vi "Result_Test.vi"(8 "error in (no error)":errorcluster caption="entrée d'erreur (pas d'erreur)", 11 "Delay en entrée":refnum<class "Enter_SN_PCRE.lvclass">) -> (0 "error out":errorcluster caption="sortie d'erreur", 3 "Delay en sortie":refnum<class "Enter_SN_PCRE.lvclass">)   [LabVIEW 2020, in "Library Test.lvlib" / "Enter_SN_PCRE.lvclass"]
uses:
  Enter_SN_PCRE.lvclass
  C:/Users/ngarcin/OneDrive - Altyor/Standard TB/Suite TB45/Class/Test/Test (Default)/Test (Default).lvclass
  Commun VI/TypeDef/Variable Printable.ctl
  Creation_SN/Creation_SN Database (Default)/Creation_SN Database (Default).lvclass
  Test_Without_Instr/Test_Without_Inst.lvclass
  Commun VI/Library Commun.lvlib
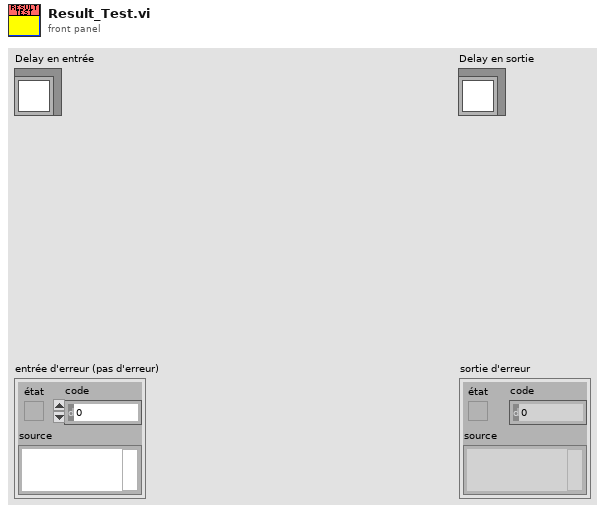
[diagram p1: front panel]
types:
  T1 = typedef "Variable Printable.ctl" = string
  T2 = enum16{"Get Variable", "Get All Variables", "Set Variable", "Delete Variable", "Delete All Variable"}
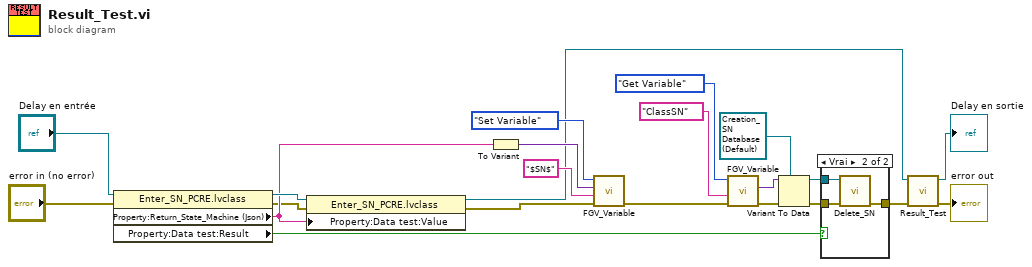
[diagram p0: block diagram]
diagram:
  n1 = property class="Enter_SN_PCRE.lvclass"(reference="Delay en entrée", error in="error in (no error)") -> (reference out=w15:refnum<class "Enter_SN_PCRE.lvclass">, error out=w12:errorcluster, "Property:Return_State_Machine (Json)"=w14:string, "Property:Data test:Result"=w1:bool)
  n2 = property class="Enter_SN_PCRE.lvclass"(reference=w15, error in=w12, "Property:Data test:Value"=w14) -> (reference out=w13:refnum<class "Enter_SN_PCRE.lvclass">, error out=w11:errorcluster)
  n3 = To Variant(anything=w14) -> (Variant=w17:variant)
  n4 = call "FGV_Variable.vi"("error in (no error)"=w11, "Variable"="$SN$" ("Name"), "Data In"=w17, "Function"=T2."Set Variable") -> ("error out"=w8:errorcluster)  [unwired: 5 in, 2 out]
  n5 = call "FGV_Variable.vi"("error in (no error)"=w8, "Variable"=T1 "ClassSN", "Function"=T2."Get Variable") -> ("error out"=w6:errorcluster, "Data Out"=w7:variant)  [unwired: 6 in, 1 out]
  n6 = Variant To Data(error in=w6, type=refnum<class "Creation_SN Database (Default).lvclass"> refnum ("Library Creation_SN.lvlib:Creation_SN Database (Default).lvclass"), Variant=w7) -> (data=w3:refnum<class "Creation_SN Database (Default).lvclass">, error out=w4:errorcluster)
  n7 = case shown="Vrai" w1 {
    tunnel: w4 -> [w23 w26]
    tunnel: w3 -> [_ w25]
    tunnel: [w23 w24] -> w2
    frame False {
    }
    frame True {
      n8 = call-dynamic "Delete_SN.vi"("error in (no error)"=w26, "Class Creation_SN (Default) en entrée"=w25) -> ("error out"=w24:errorcluster)  [unwired: 8 in, 1 out]
    }
  }
  n9 = call-parent "Result_Test.vi"("error in (no error)"=w2, "Test_Without_Inst en entrée"=w13) -> ("error out"=→"error out":errorcluster, "Test_Without_Inst en sortie"=→"Delay en sortie":refnum<class "Enter_SN_PCRE.lvclass">)  [unwired: 8 in]
